vi "ControlServo.vi"(0 "position":u8(slide) scale=125.0..230.0) -> ()   [LabVIEW 2014]
uses:
  <vilib>/Instr/_visa.llb/VISA Configure Serial Port (Instr).vi
panel:
  in  "servo #":u8
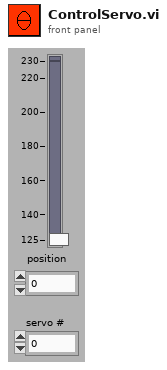
[diagram p1: front panel]
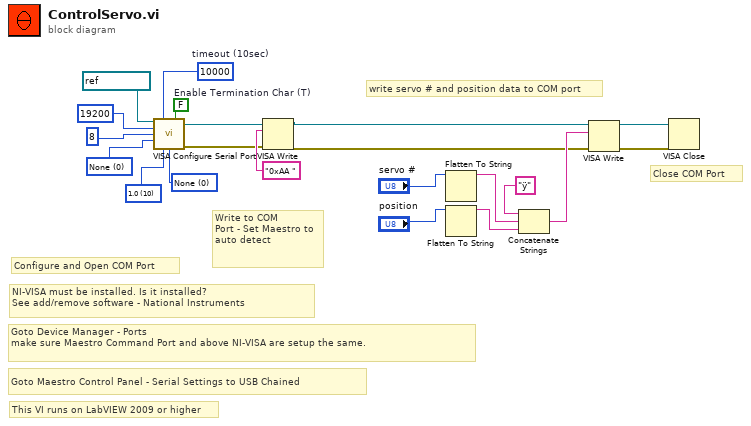
[diagram p0: block diagram]
diagram:
  w13 = u16 0 items=["None"=0, "XON/XOFF"=1, "RTS/CTS"=2, "DTR/DSR"=4] ("flow control")
  w14 = u16 10 items=["1.0"=10, "1.5"=15, "2.0"=20] ("stop bits")
  w15 = u16 0 items=["None", "Odd", "Even", "Mark", "Space"] ("parity")
  w19 = FALSE  # Enable Termination Char (T)
  w20 = u32 10000  # timeout (10sec)
  # "write servo # and position data to COM port"
  # "This VI runs on LabVIEW 2009 or higher"
  # "Goto Maestro Control Panel - Serial Settings to USB Chained"
  # "Close COM Port"
  # "Configure and Open COM Port"
  # "Goto Device Manager - Ports \nmake sure Maestro Command Port and above NI-VISA are setup the same."
  # "NI-VISA must be installed. Is it installed?\nSee add/remove software - National Instruments"
  # "Write to COM \nPort - Set Maestro to auto detect"
  n1 = call-poly "VISA Configure Serial Port"("VISA resource name"=refnum<visa-resource-name> "COM10", "timeout (10sec)"=w20, "Enable Termination\nChar (T)"=w19, "baud rate (9600)"=u32 19200 ("baud rate"), "data bits (8)"=u16 8 ("data bits"), "parity (0:none)"=w15, "stop bits (10: 1 bit)"=w14, "flow control (0:none)"=w13) -> ("VISA resource name out"=w11:refnum<visa-resource-name>, "error out"=w12:errorcluster)  [unwired: 1 in, 5 out]
  n2 = VISA Write(VISA resource name=w11, write buffer="0xAA ", error in (no error)=w12) -> (VISA resource name out=w1:refnum<visa-resource-name>, error out=w2:errorcluster)  [unwired: 1 out]
  n3 = Flatten To String(anything="servo #") -> (data string=w6:string)  [unwired: 1 in, 4 out]
  n4 = Flatten To String(anything="position") -> (data string=w7:string)  [unwired: 1 in, 4 out]
  n5 = Concatenate Strings("ÿ", w6, w7) -> (w8:string)
  n6 = VISA Write(VISA resource name=w1, write buffer=w8, error in (no error)=w2) -> (VISA resource name out=w4:refnum<visa-resource-name>, error out=w3:errorcluster)  [unwired: 1 out]
  n7 = VISA Close(VISA resource name=w4, error in (no error)=w3) -> ()  [unwired: 1 out]
